vi "PH_Cam_BaseClass.pack PSDB Data.vi"(0 "VI in":refnum<vi>, 5 "error in (no error)":errorcluster) -> (14 "VI out":refnum<vi>, 16 "PSDB Image Data Array":T2[](array[typedef]), 17 "PSDB String Data Array":T1[](array[typedef]), 19 "error out":errorcluster)   [LabVIEW 2014, in "PH_Cam_BaseClass.lvlib"]
doc: "This VI packs data for the PHELIX shot data base."
uses:
  PH_Cam_BaseClass.lvlib
  PH_PSDBWriter/PH_PSDBWriter.Image dataset.ctl
  <vilib>/vision/Image Controls.llb/IMAQ Image.ctl
  PH_PSDBWriter/PH_PSDBWriter.String dataset.ctl
  PH_PSDBWriter/PH_PSDBWriter.lvlib
  PH_StatusHandler/PH_StatusHandler.lvlib
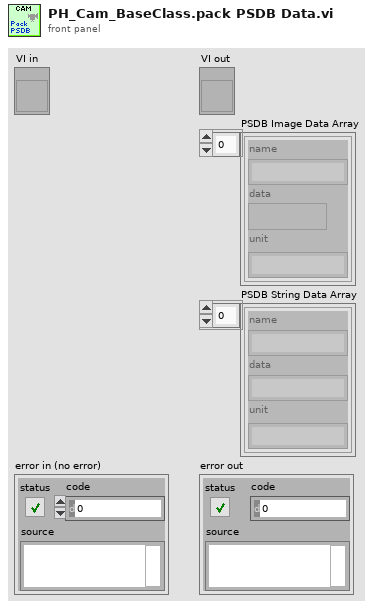
[diagram p1: front panel]
types:
  T1 = typedef "PH_PSDBWriter.lvlib/PH_PSDBWriter.String dataset.ctl" = cluster{"name":string, "data":string, "unit":string}
  T2 = typedef "PH_PSDBWriter.lvlib/PH_PSDBWriter.Image dataset.ctl" = cluster{"name":string, "data":T3, "unit":string}
  T3 = typedef "IMAQ Image.ctl" = refnum<image>
  T4 = typedef "PH_Cam_BaseClass.lvlib/PH_Cam_BaseClass.i attribute.ctl" = cluster{"Gui Refs":T5, "Cam":cluster{"Source Notifier":refnum<notifier>, "Error":errorcluster, "Camera ID":string}, "Images":cluster{"Cam":T3, "Operation":T3, "PSDB":T3}, "Window Image":cluster{"Indicate Image":bool, "Window No.":i32, "Scale Facor":dbl, "Center Cross":bool, "Subtract Backgr":bool, "CoG":bool, "Color Palette":cluster{"Red":u8, "Green":u8, "Blue":u8}[], "Image On":bool}, "Default Prdc Int":i32, "Performance":cluster{"on":bool, "Timestamp Last Frame":i32}, "Histogram":cluster{"on":bool, "Mapping":bool}, "Save Image":cluster{"Save":bool, "File refnum":refnum<file>}, "Setting Service ID":i32, "Screen":cluster{"x-resolution":i16, "y-resolution":i16}, "On":bool, "Constructor finished":bool, "configured":bool}
  T5 = typedef "PH_Cam_BaseClass.lvlib/PH_Cam_BaseClass.GUI Refs.ctl" = cluster{"Frame Rate":refnum<vi>, "Get Frame Rate":refnum<vi>, "Show Image":refnum<vi>, "Get Histogram":refnum<vi>, "Mapping":refnum<vi>, "Histogram":refnum<vi>, "Center Cross":refnum<vi>, "Center of Gravity":refnum<vi>, "Scale Factor [%]":refnum<vi>, "Save Image":refnum<vi>, "Palette":refnum<vi>, "Subtract Background":refnum<vi>, "Cam Error":refnum<vi>, "On":refnum<vi>, "Cam List":refnum<vi>}
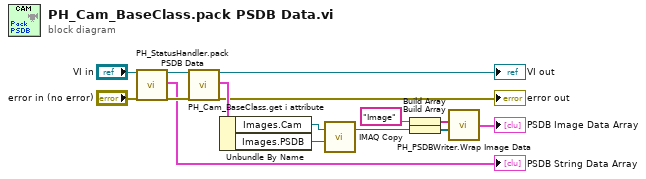
[diagram p0: block diagram]
diagram:
  n1 = call "PH_StatusHandler.pack PSDB Data.vi"("VI in"="VI in", "error in (no error)"="error in (no error)") -> ("VI out"=w4:refnum<vi>, "PSDB String Data Array"=→"PSDB String Data Array":T1[], "error out"=w2:errorcluster)  [unwired: 15 in]
  n2 = call "PH_Cam_BaseClass.get i attribute.vi"("i ref in"=w4, "error in (no error)"=w2) -> ("i ref out"=→"VI out":refnum<vi>, "i attribute"=w13:T4, "error out"=→"error out":errorcluster)  [unwired: 15 in]
  n3 = Unbundle By Name(w13) -> ("Images.Cam"=w14:T3, "Images.PSDB"=w15:T3)
  n4 = call "IMAQ Copy"("Image Dst"=w15, "Image Src"=w14) -> ("Image Dst Out"=w8:T3)  [unwired: 4 in, 1 out]
  n5 = Build Array("Image" ("name")) -> (w10:string[])
  n6 = Build Array(w8) -> (w9:T3[])
  n7 = call "PH_PSDBWriter.Wrap Image Data.vi"("Data Arrray"=w9, "Name Array"=w10) -> ("PSDB Image Data Array"=→"PSDB Image Data Array":T2[])  [unwired: 2 in]
